vi "write_DACs.vi"(7 "converter box version":i16=1 min=1 max=2, 11 "DAC values in":T1 {"bit index" min=-1 max=17 step=1; "channel index" max=7 step=1; "offset" max=4095; "DAC voltage"."ch1" max=4095 step=1; "DAC voltage"."ch0" max=4095 step=1}) -> (3 "DAQ values out":T1 {"bit index" min=-1 max=17 step=1; "channel index" max=7 step=1; "offset" max=4095; "DAC voltage"."ch1" max=4095 step=1; "DAC voltage"."ch0" max=4095 step=1})   [LabVIEW 2010]
uses:
  FPGA_Typedefs/DAC_values_cluster.ctl
  FPGA_Typedefs/DAC_voltage_cluster.ctl
  <vilib>/eio/EIONode/EIONode.xnode
  <vilib>/rvi/eio/nirviEIOImplementation/nirviEIOImplementation.xnode
  <vilib>/rvi/eio/common/nirviEmuClasses.ctl
  <vilib>/rvi/eio/common/nirviEmuTemplateMethod_noerrors.vi
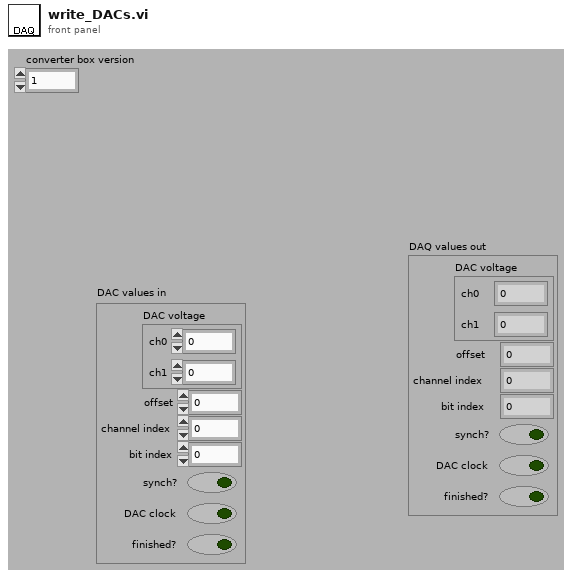
[diagram p1: front panel]
types:
  T1 = typedef "DAC_values_cluster.ctl" = cluster{"DAC voltage":T2, "offset":u16, "channel index":u16, "bit index":i32, "synch?":bool, "DAC clock":bool, "finished?":bool}
  T2 = typedef "DAC_voltage_cluster.ctl" = cluster{"ch0":u16, "ch1":u16}
  T3 = typedef "nirviEmuClasses.ctl" = enum16{"IO Read", "IO Write", "Method", "Property Read", "Property Write"}
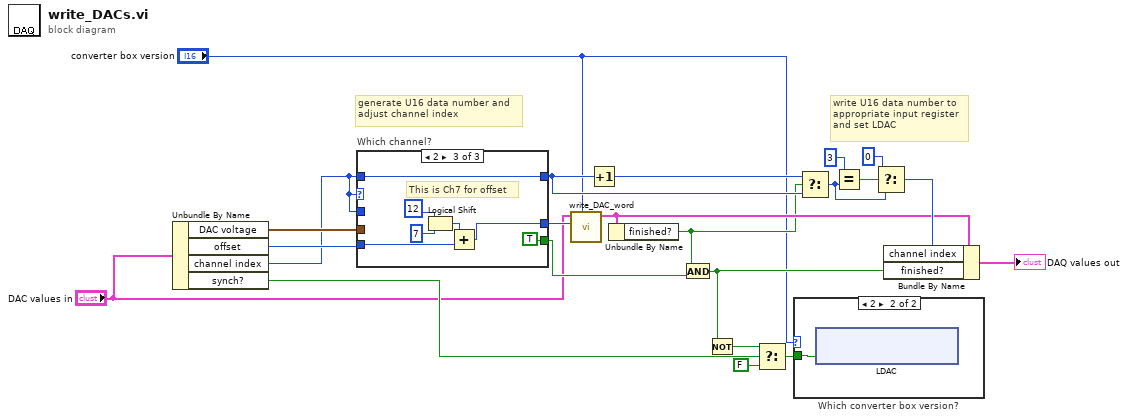
[diagram p0: block diagram]
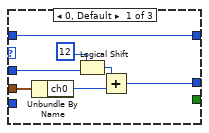
[diagram p3: hidden frame]
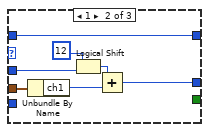
[diagram p4: hidden frame]
diagram:
  # "write U16 data number to\nappropriate input register\nand set LDAC"
  # "generate U16 data number and\nadjust channel index"
  n1 = Unbundle By Name("DAC values in") -> ("DAC voltage"=w11:T2, "offset"=w10:u16, "channel index"=w1:u16, "synch?"=w9:bool)
  n2 = case "Which channel?" shown="2" w1 {
    tunnel: w11 -> [w25 w36 _]
    tunnel: w10 -> [_ _ w41]
    tunnel: w1 -> [w26 w33 _]
    tunnel: [w23 w30 w39] -> w22
    tunnel: [_ _ TRUE] -> w19
    tunnel: w1 -> [w24 w31 w37]
    tunnel: [w24 w31 w37] -> w17
    frame 0, Default {
      n3 = Unbundle By Name(w25) -> ("ch0"=w29:u16)
      n4 = Logical Shift(y=u16 12, x=w26) -> (x << y=w27:u16)
      n5 = Add(x=w27, y=w29) -> (x+y=w23:u16)
    }
    frame 1 {
      n6 = Unbundle By Name(w36) -> ("ch1"=w32:u16)
      n7 = Logical Shift(y=u16 12, x=w33) -> (x << y=w35:u16)
      n8 = Add(x=w35, y=w32) -> (x+y=w30:u16)
    }
    frame 2 {
      # "This is Ch7 for offset"
      n9 = Logical Shift(y=u16 12, x=u16 7) -> (x << y=w42:u16)
      n10 = Add(x=w42, y=w41) -> (x+y=w39:u16)
    }
  }
  n11 = call "write_DAC_word.vi"("converter box version"="converter box version", "U16 data number"=w22, "DAC values in"="DAC values in") -> ("DAC values out"=w4:T1)  [unwired: 8 in]
  n12 = Increment(x=w17) -> (x+1=w16:u16)
  n13 = Unbundle By Name(w4) -> ("finished?"=w3:bool)
  n14 = And(x=w3, y=w19) -> (x .and. y?=w8:bool)
  n15 = Not(x=w8) -> (.not. x?=w18:bool)
  n16 = Select(t=w18, s=w9, f=FALSE) -> (s? t:f=w20:bool)
  n17 = case "Which converter box version?" shown="2" "converter box version" {
    tunnel: w20 -> [_ w44]
    frame Default {
    }
    frame 2 {
      n18 = xnode "LDAC"("Connector1/DIO32"=w44) -> ()  [unwired: 1 in, 1 out]
    }
  }
  n19 = Select(t=w16, s=w3, f=w17) -> (s? t:f=w12:u16)
  n20 = Equal?(x=u16 3, y=w12) -> (x = y?=w14:bool)
  n21 = Select(t=u16 0, s=w14, f=w12) -> (s? t:f=w7:u16)
  n22 = Bundle By Name(cluster=w4, "channel index"=w7, "finished?"=w8) -> (→"DAQ values out":T1)
